vi "CRYUnflatten Statistic.vi"(11 "Flatten Statistics":string) -> (0 "Error?":bool, 2 "Statistics":T1, 3 "Header info":T2={"Data type"="Data            ", "Version"=1, "Dimensions"=0})   [LabVIEW 2013]
uses:
  Typedef Control/CRYStatistic cluster.ctl
panel:
  in  "error in (no error)":errorcluster
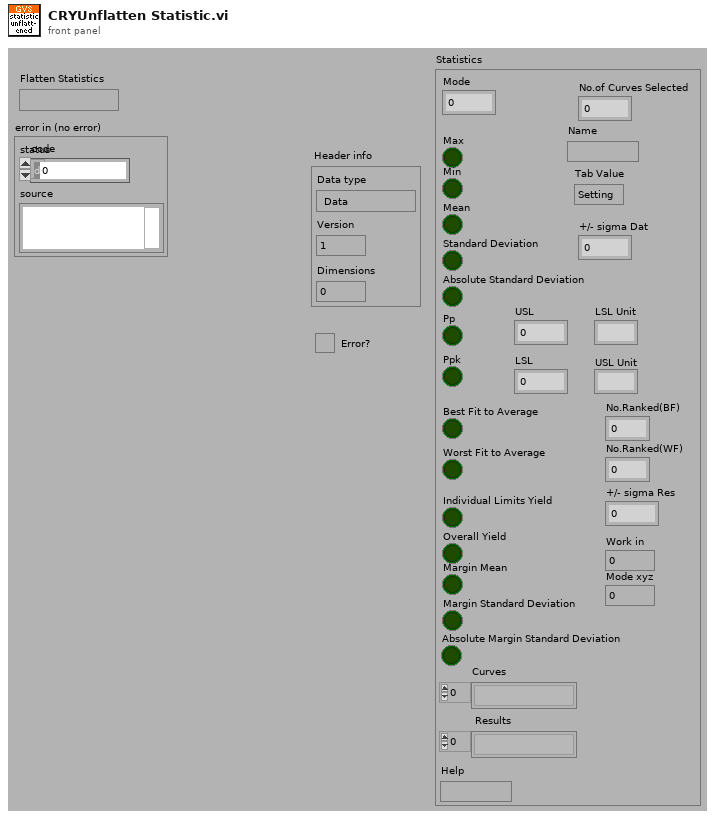
[diagram p1: front panel]
types:
  T1 = typedef "CRYStatistic cluster.ctl" = cluster{"Mode":u16, "No.Ranked(BF)":i32, "No.Ranked(WF)":i32, "Absolute Margin Standard Deviation":bool, "+/- sigma Res":i32, "Margin Standard Deviation":bool, "Margin Mean":bool, "Overall Yield":bool, "Individual Limits Yield":bool, "LSL Unit":string, "USL Unit\n":string, "LSL":dbl, "USL":dbl, "Worst Fit to Average":bool, "Best Fit to Average":bool, "Ppk":bool, "Pp":bool, "Absolute Standard Deviation":bool, "+/- sigma Dat":i32, "Standard Deviation ":bool, "Mean":bool, "Min ":bool, "Max ":bool, "No.of Curves Selected":i32, "Curves":string[], " Results":string[], "Name":string, "Help":string, "Tab Value":enum32{"Setting", "Help"}, "Work in":u16, "Mode xyz":u16}
  T2 = cluster{"Data type":string, "Version":u16, "Dimensions":u8}
  T3 = cluster{"Mode":u16, "No.Ranked(BF)":i32, "No.Ranked(WF)":i32, "Absolute Margin Standard Deviation":bool, "+/- sigma Res":i32, "Margin Standard Deviation":bool, "Margin Mean":bool, "Overall Yield":bool, "Individual Limits Yield":bool, "LSL Unit":string, "USL Unit\n":string, "LSL":dbl, "USL":dbl, "Worst Fit to Average":bool, "Best Fit to Average":bool, "Ppk":bool, "Pp":bool, "Absolute Standard Deviation":bool, "+/- sigma Dat":i32, "Standard Deviation ":bool, "Mean":bool, "Min ":bool, "Max ":bool, "No.of Curves Selected":i32, "Curves":string[], " Results":string[], "Name":string, "Help":string, "Tab Value":enum32{"Setting", "Help"}, "Work in":u16, "Mode xyz":u16}
  T4 = cluster{"unsigned byte array[0]":u8, "unsigned byte array[1]":u8, "unsigned byte array[2]":u8}
  T5 = cluster{"Mode":u16, "No.Ranked(BF)":i32, "No.Ranked(WF)":i32, "Absolute Margin Standard Deviation":bool, "+/- sigma Res":i32, "Margin Standard Deviation":bool, "Margin Mean":bool, "Overall Yield":bool, "Individual Limits Yield":bool, "LSL Unit":string, "USL Unit\n":string, "LSL":i32, "USL":i32, "Worst Fit to Average":bool, "Best Fit to Average":bool, "Ppk":bool, "Pp":bool, "Absolute Standard Deviation":bool, "+/- sigma Dat":i32, "Standard Deviation ":bool, "Mean":bool, "Min ":bool, "Max ":bool, "No.of Curves Selected":i32, "Curves":string[], " Results":string[], "Name":string}
  T6 = cluster{"Mode":u16, "No.Ranked(BF)":i32, "No.Ranked(WF)":i32, "Absolute Margin Standard Deviation":bool, "+/- sigma Res":i32, "Margin Standard Deviation":bool, "Margin Mean":bool, "Overall Yield":bool, "Individual Limits Yield":bool, "LSL Unit":string, "USL Unit\n":string, "LSL":dbl, "USL":dbl, "Worst Fit to Average":bool, "Best Fit to Average":bool, "Ppk":bool, "Pp":bool, "Absolute Standard Deviation":bool, "+/- sigma Dat":i32, "Standard Deviation ":bool, "Mean":bool, "Min ":bool, "Max ":bool, "No.of Curves Selected":i32, "Curves":string[], " Results":string[], "Name":string, "Help":string, "Tab Value":enum32{"Setting", "Help"}}
  T7 = cluster{"substring":string, u16, "unsigned byte array[2]":u8}
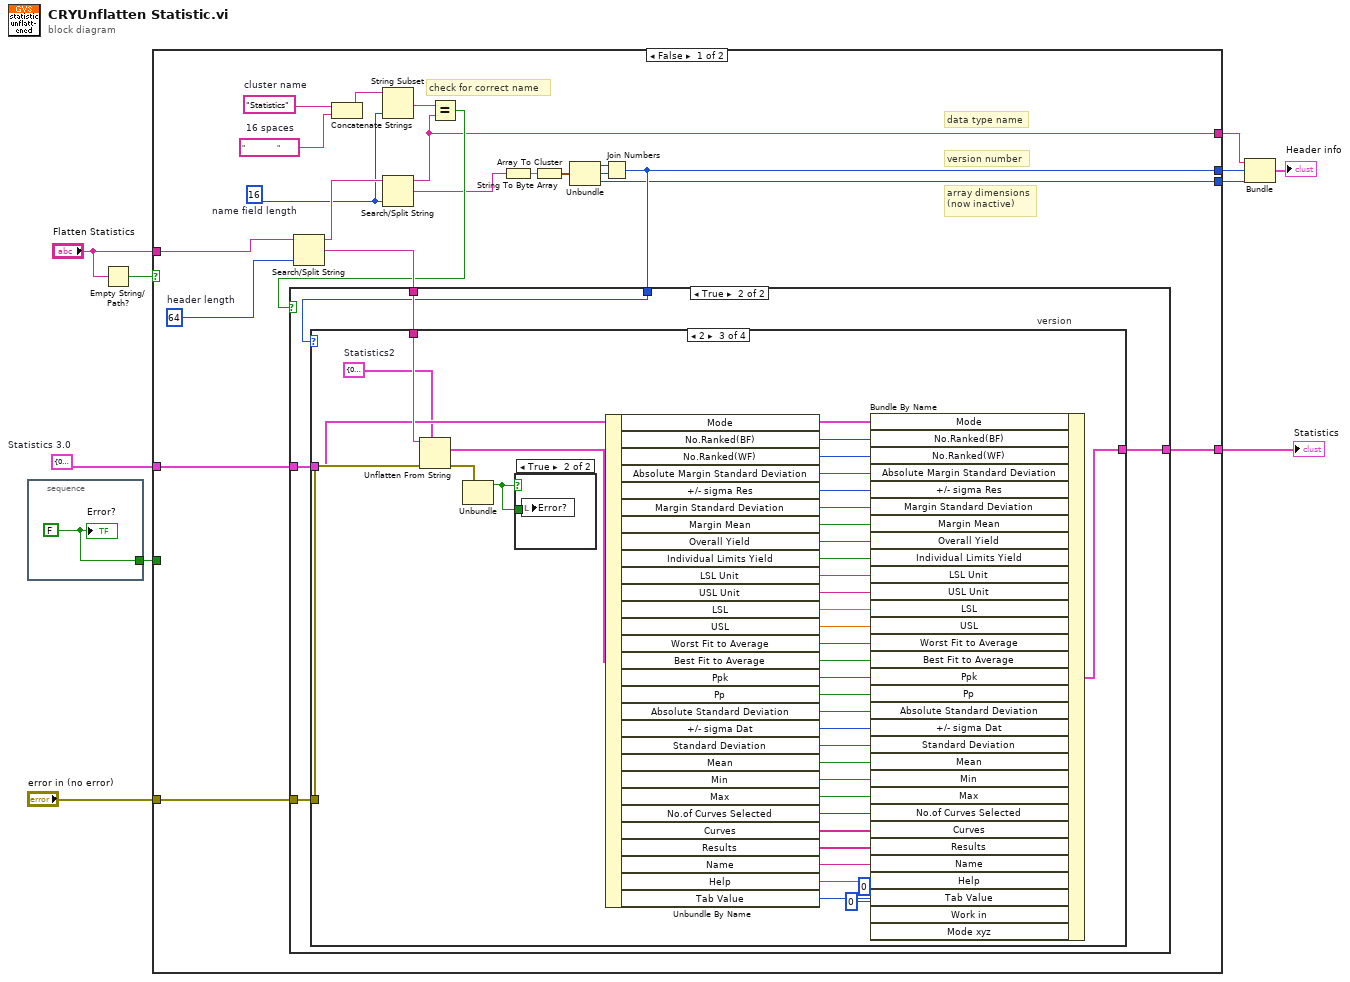
[diagram p0: block diagram]
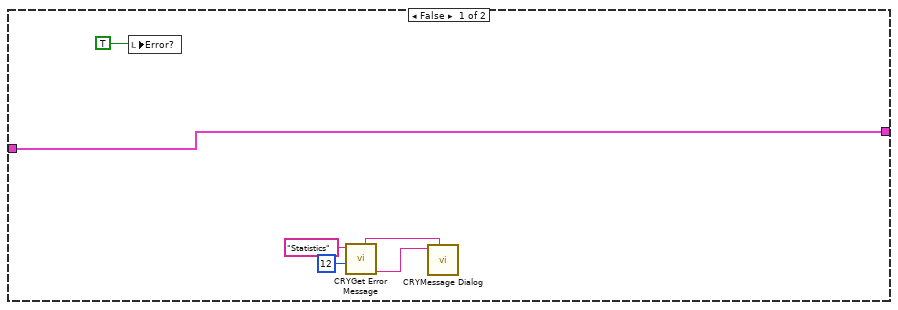
[diagram p2: hidden frame]
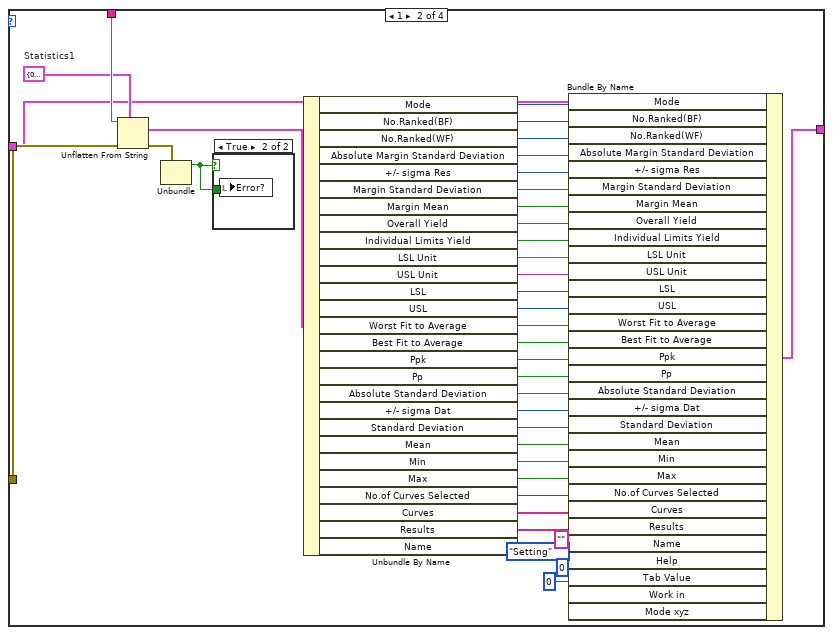
[diagram p4: hidden frame]
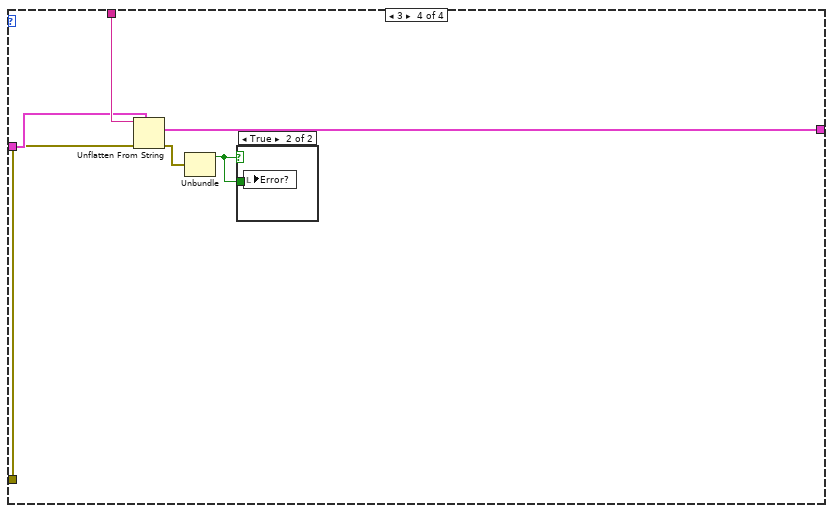
[diagram p7: hidden frame]
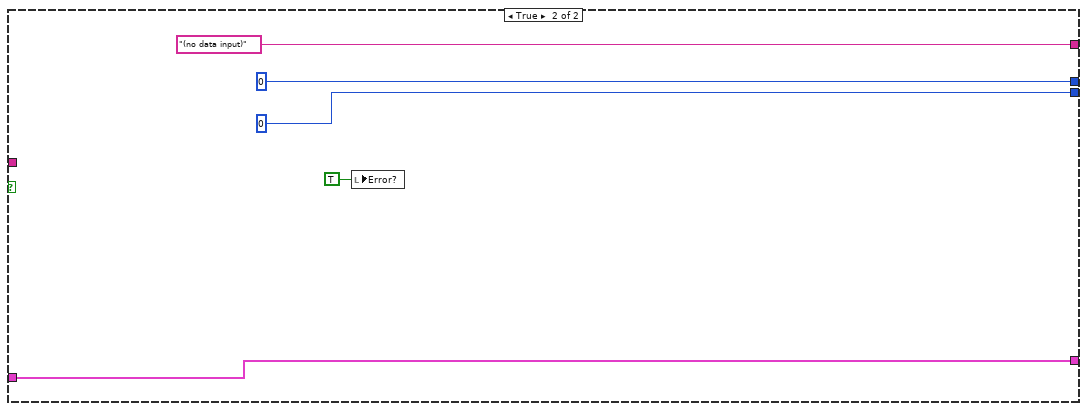
[diagram p9: hidden frame]
diagram:
  w2 = T3 {"Mode"=0, "No.Ranked(BF)"=0, "No.Ranked(WF)"=0, "Absolute Margin Standard Deviation"=FALSE, "+/- sigma Res"=0, "Margin Standard Deviation"=FALSE, "Margin Mean"=FALSE, "Overall Yield"=FALSE, "Individual Limits Yield"=FALSE, "LSL Unit"="", "USL Unit\n"="", "LSL"=0.0, "USL"=0.0, "Worst Fit to Average"=FALSE, "Best Fit to Average"=FALSE, "Ppk"=FALSE, "Pp"=FALSE, "Absolute Standard Deviation"=FALSE, "+/- sigma Dat"=0, "Standard Deviation "=FALSE, "Mean"=FALSE, "Min "=FALSE, "Max "=FALSE, "No.of Curves Selected"=0, "Curves"=[], " Results"=[], "Name"="", "Help"="", "Tab Value"=enum."Setting", "Work in"=0, "Mode xyz"=0}  # Statistics 3.0
  n1 = stacked-sequence {
    tunnel: [w11] -> w5
    frame #0 {
      w11 = FALSE
      "Error?" <- w11
    }
  }
  n2 = Empty String/Path?(string/path="Flatten Statistics") -> (empty?=w10:bool)
  n3 = case shown="False" w10 {
    tunnel: "Flatten Statistics" -> [w32 _]
    tunnel: [w24 u16 0] -> w8
    tunnel: [w16 u8 0] -> w9
    tunnel: [w17 "(no data input)" ("substring")] -> w7
    tunnel: w5 -> [_ _]
    tunnel: [w15 w132] -> w1
    tunnel: w2 -> [w14 w132]
    tunnel: "error in (no error)" -> [w13 _]
    frame False {
      w12 = 64  # header length
      w21 = "                "  # 16 spaces
      w22 = "Statistics"  # cluster name
      w19 = 16  # name field length
      # "check for correct name"
      # "array dimensions\n(now inactive)"
      # "version number"
      # "data type name"
      n4 = Search/Split String(string=w32, offset (0)=w12) -> (substring before match=w26:string, match + rest of string=w27:string)  [unwired: 2 out]
      n5 = Concatenate Strings(w22, w21) -> (w20:string)
      n6 = String Subset(string=w20, length (rest)=w19) -> (substring=w18:string)  [unwired: 1 out]
      n7 = Search/Split String(string=w26, offset (0)=w19) -> (substring before match=w17:string, match + rest of string=w23:string)  [unwired: 2 out]
      n8 = Equal?(x=w18, y=w17) -> (x = y?=w25:bool)
      n9 = String To Byte Array(string=w23) -> (unsigned byte array=w31:u8[])
      n10 = Array To Cluster(array=w31) -> (cluster=w30:T4)
      n11 = Unbundle(w30) -> ("unsigned byte array[0]"=w29:u8, "unsigned byte array[1]"=w28:u8, "unsigned byte array[2]"=w16:u8)
      n12 = Join Numbers(hi=w29, lo=w28) -> ((hi.lo)=w24:u16)
      n13 = case shown="True" w25 {
        tunnel: w27 -> [_ w43]
        tunnel: w24 -> [_ w42]
        tunnel: [w37 w41] -> w15
        tunnel: w14 -> [w37 w40]
        tunnel: w13 -> [_ w39]
        frame False {
          n14 = local write "Error?"(TRUE) -> ()
          n15 = call "CRYGet Error Message.vi"("Error No"=12 ("No"), "Kind"="Statistics") -> ("Message Sub 3"=w33:string, "Window Title"=w34:string)  [unwired: 4 in, 4 out]
          n16 = call "CRYMessage Dialog.vi"("Window Title"=w34, "Message Content"=w33) -> ()  [unwired: 8 in, 2 out]
        }
        frame True {
          n17 = case "version" shown="2" w42 {
            tunnel: w43 -> [_ w83 w123 w130]
            tunnel: [w44 w75 w117 w127] -> w41
            tunnel: w40 -> [w44 w77 w118 w128]
            tunnel: w39 -> [_ w80 w120 w125]
            frame Default {
            }
            frame 1 {
              w79 = T5 {"Mode"=0, "No.Ranked(BF)"=0, "No.Ranked(WF)"=0, "Absolute Margin Standard Deviation"=FALSE, "+/- sigma Res"=0, "Margin Standard Deviation"=FALSE, "Margin Mean"=FALSE, "Overall Yield"=FALSE, "Individual Limits Yield"=FALSE, "LSL Unit"="", "USL Unit\n"="", "LSL"=0, "USL"=0, "Worst Fit to Average"=FALSE, "Best Fit to Average"=FALSE, "Ppk"=FALSE, "Pp"=FALSE, "Absolute Standard Deviation"=FALSE, "+/- sigma Dat"=0, "Standard Deviation "=FALSE, "Mean"=FALSE, "Min "=FALSE, "Max "=FALSE, "No.of Curves Selected"=0, "Curves"=[], " Results"=[], "Name"=""}  # Statistics1
              n18 = Unflatten From String(type=w79, binary string=w83, error in (no error)=w80) -> (value=w78:T5, error out=w81:errorcluster)  [unwired: 3 out]
              n19 = Unbundle(w81) -> ("status"=w82:bool)  [unwired: 2 out]
              n20 = case shown="True" w82 {
                tunnel: w82 -> [_ w84]
                frame False {
                }
                frame True {
                  n21 = local write "Error?"(w84) -> ()
                }
              }
              n22 = Unbundle By Name(w78) -> ("Mode"=w74:u16, "No.Ranked(BF)"=w73:i32, "No.Ranked(WF)"=w72:i32, "Absolute Margin Standard Deviation"=w71:bool, "+/- sigma Res"=w70:i32, "Margin Standard Deviation"=w69:bool, "Margin Mean"=w68:bool, "Overall Yield"=w67:bool, "Individual Limits Yield"=w66:bool, "LSL Unit"=w65:string, "USL Unit"=w64:string, "LSL"=w63:i32, "USL"=w62:i32, "Worst Fit to Average"=w61:bool, "Best Fit to Average"=w60:bool, "Ppk"=w59:bool, "Pp"=w58:bool, "Absolute Standard Deviation"=w57:bool, "+/- sigma Dat"=w56:i32, "Standard Deviation"=w55:bool, "Mean"=w54:bool, "Min"=w53:bool, "Max"=w52:bool, "No.of Curves Selected"=w51:i32, "Curves"=w50:string[], "Results"=w49:string[], "Name"=w48:string)
              n23 = Bundle By Name(cluster=w77, "Mode"=w74, "No.Ranked(BF)"=w73, "No.Ranked(WF)"=w72, "Absolute Margin Standard Deviation"=w71, "+/- sigma Res"=w70, "Margin Standard Deviation"=w69, "Margin Mean"=w68, "Overall Yield"=w67, "Individual Limits Yield"=w66, "LSL Unit"=w65, "USL Unit"=w64, "LSL"=w63, "USL"=w62, "Worst Fit to Average"=w61, "Best Fit to Average"=w60, "Ppk"=w59, "Pp"=w58, "Absolute Standard Deviation"=w57, "+/- sigma Dat"=w56, "Standard Deviation"=w55, "Mean"=w54, "Min"=w53, "Max"=w52, "No.of Curves Selected"=w51, "Curves"=w50, "Results"=w49, "Name"=w48, "Help"="", "Tab Value"=enum32{"Setting", "Help"}."Setting", "Work in"=u16 0, "Mode xyz"=u16 0) -> (w75:T3)
            }
            frame 2 {
              w89 = T6 {"Mode"=0, "No.Ranked(BF)"=0, "No.Ranked(WF)"=0, "Absolute Margin Standard Deviation"=FALSE, "+/- sigma Res"=0, "Margin Standard Deviation"=FALSE, "Margin Mean"=FALSE, "Overall Yield"=FALSE, "Individual Limits Yield"=FALSE, "LSL Unit"="", "USL Unit\n"="", "LSL"=0.0, "USL"=0.0, "Worst Fit to Average"=FALSE, "Best Fit to Average"=FALSE, "Ppk"=FALSE, "Pp"=FALSE, "Absolute Standard Deviation"=FALSE, "+/- sigma Dat"=0, "Standard Deviation "=FALSE, "Mean"=FALSE, "Min "=FALSE, "Max "=FALSE, "No.of Curves Selected"=0, "Curves"=[], " Results"=[], "Name"="", "Help"="", "Tab Value"=enum."Setting"}  # Statistics2
              n24 = Unflatten From String(type=w89, binary string=w123, error in (no error)=w120) -> (value=w119:T6, error out=w121:errorcluster)  [unwired: 3 out]
              n25 = Unbundle(w121) -> ("status"=w122:bool)  [unwired: 2 out]
              n26 = case shown="True" w122 {
                tunnel: w122 -> [_ w124]
                frame False {
                }
                frame True {
                  n27 = local write "Error?"(w124) -> ()
                }
              }
              n28 = Unbundle By Name(w119) -> ("Mode"=w116:u16, "No.Ranked(BF)"=w115:i32, "No.Ranked(WF)"=w114:i32, "Absolute Margin Standard Deviation"=w113:bool, "+/- sigma Res"=w112:i32, "Margin Standard Deviation"=w111:bool, "Margin Mean"=w110:bool, "Overall Yield"=w109:bool, "Individual Limits Yield"=w108:bool, "LSL Unit"=w107:string, "USL Unit"=w106:string, "LSL"=w105:dbl, "USL"=w104:dbl, "Worst Fit to Average"=w103:bool, "Best Fit to Average"=w102:bool, "Ppk"=w101:bool, "Pp"=w100:bool, "Absolute Standard Deviation"=w99:bool, "+/- sigma Dat"=w98:i32, "Standard Deviation"=w97:bool, "Mean"=w96:bool, "Min"=w95:bool, "Max"=w94:bool, "No.of Curves Selected"=w93:i32, "Curves"=w92:string[], "Results"=w91:string[], "Name"=w90:string, "Help"=w88:string, "Tab Value"=w87:enum32{"Setting", "Help"})
              n29 = Bundle By Name(cluster=w118, "Mode"=w116, "No.Ranked(BF)"=w115, "No.Ranked(WF)"=w114, "Absolute Margin Standard Deviation"=w113, "+/- sigma Res"=w112, "Margin Standard Deviation"=w111, "Margin Mean"=w110, "Overall Yield"=w109, "Individual Limits Yield"=w108, "LSL Unit"=w107, "USL Unit"=w106, "LSL"=w105, "USL"=w104, "Worst Fit to Average"=w103, "Best Fit to Average"=w102, "Ppk"=w101, "Pp"=w100, "Absolute Standard Deviation"=w99, "+/- sigma Dat"=w98, "Standard Deviation"=w97, "Mean"=w96, "Min"=w95, "Max"=w94, "No.of Curves Selected"=w93, "Curves"=w92, "Results"=w91, "Name"=w90, "Help"=w88, "Tab Value"=w87, "Work in"=u16 0, "Mode xyz"=u16 0) -> (w117:T3)
            }
            frame 3 {
              n30 = Unflatten From String(type=w128, binary string=w130, error in (no error)=w125) -> (value=w127:T3, error out=w126:errorcluster)  [unwired: 3 out]
              n31 = Unbundle(w126) -> ("status"=w129:bool)  [unwired: 2 out]
              n32 = case shown="True" w129 {
                tunnel: w129 -> [_ w131]
                frame False {
                }
                frame True {
                  n33 = local write "Error?"(w131) -> ()
                }
              }
            }
          }
        }
      }
    }
    frame True {
      n34 = local write "Error?"(TRUE ("Error?")) -> ()
    }
  }
  "Statistics" <- w1
  n35 = Bundle("substring"=w7, w8, "unsigned byte array[2]"=w9) -> (→"Header info":T7)  [unwired: 1 out]
